vi "spike_data_packete.vi"(8 "Log File in":refnum<k34>, 11 "data out":string) -> (3 "output cluster":T1)   [LabVIEW 2017]
uses:
  Control 2.ctl
panel:
  out "data":string
  in  "?":T1
  out "DIN":string
  out "DEV":string
  out "RES":string
  out "LEN":string
  out "SYNC":string
  out "CMD":string
  out "A(I16) 11":i16
  out "Received Data 4":dbl[](graph)
  out "Received Data 3":T2(graph)
  out "BR4_5 (bending Y) 5":string
  out "BR3_5 (bending X) 5":string
  out "BR4_7 (bending Y) 7":string
  out "BR3_7 (bending X) 7":string
  out "BR2_7 (torsion)6 2":string
  out "BR1_7 (axial_force_ 7":string
  out "BR4_6 (bending Y) 6":string
  out "BR3_6 (bending X) 6":string
  out "BR2_6 (torsion)6":string
  out "BR1_6 (axial_force_ 6":string
  out "BR2_5 (torsion) 5":string
  out "BR1_5 (axial_force_ 5":string
  out "BR4_4 (bending Y) 4":string
  out "BR3_4 (bending X) 4":string
  out "BR2_4 (torsion) 4":string
  out "BR1_4 (axial_force_ 4":string
  out "BR4_3 (bending Y) 3":string
  out "BR3_3 (bending X) 3":string
  out "BR2_3 (torsion) 3":string
  out "BR1_3 (axial_force_ 3":string
  out "BR4_2 (bending Y) 2":string
  out "BR3_2 (bending X) 2":string
  out "RSSI":string
  out "PKT":string
  out "SPEF":string
  out "SPER":string
  out "BR2_2 (torsion) 2":string
  out "BR1_2 (axial_force_ 2":string
  out "BR4_1 (bending Y)":string
  out "BR3_1 (bending X)":string
  out "BR2_1 (torsion)":string
  out "BR1_1 (axial_force_":string
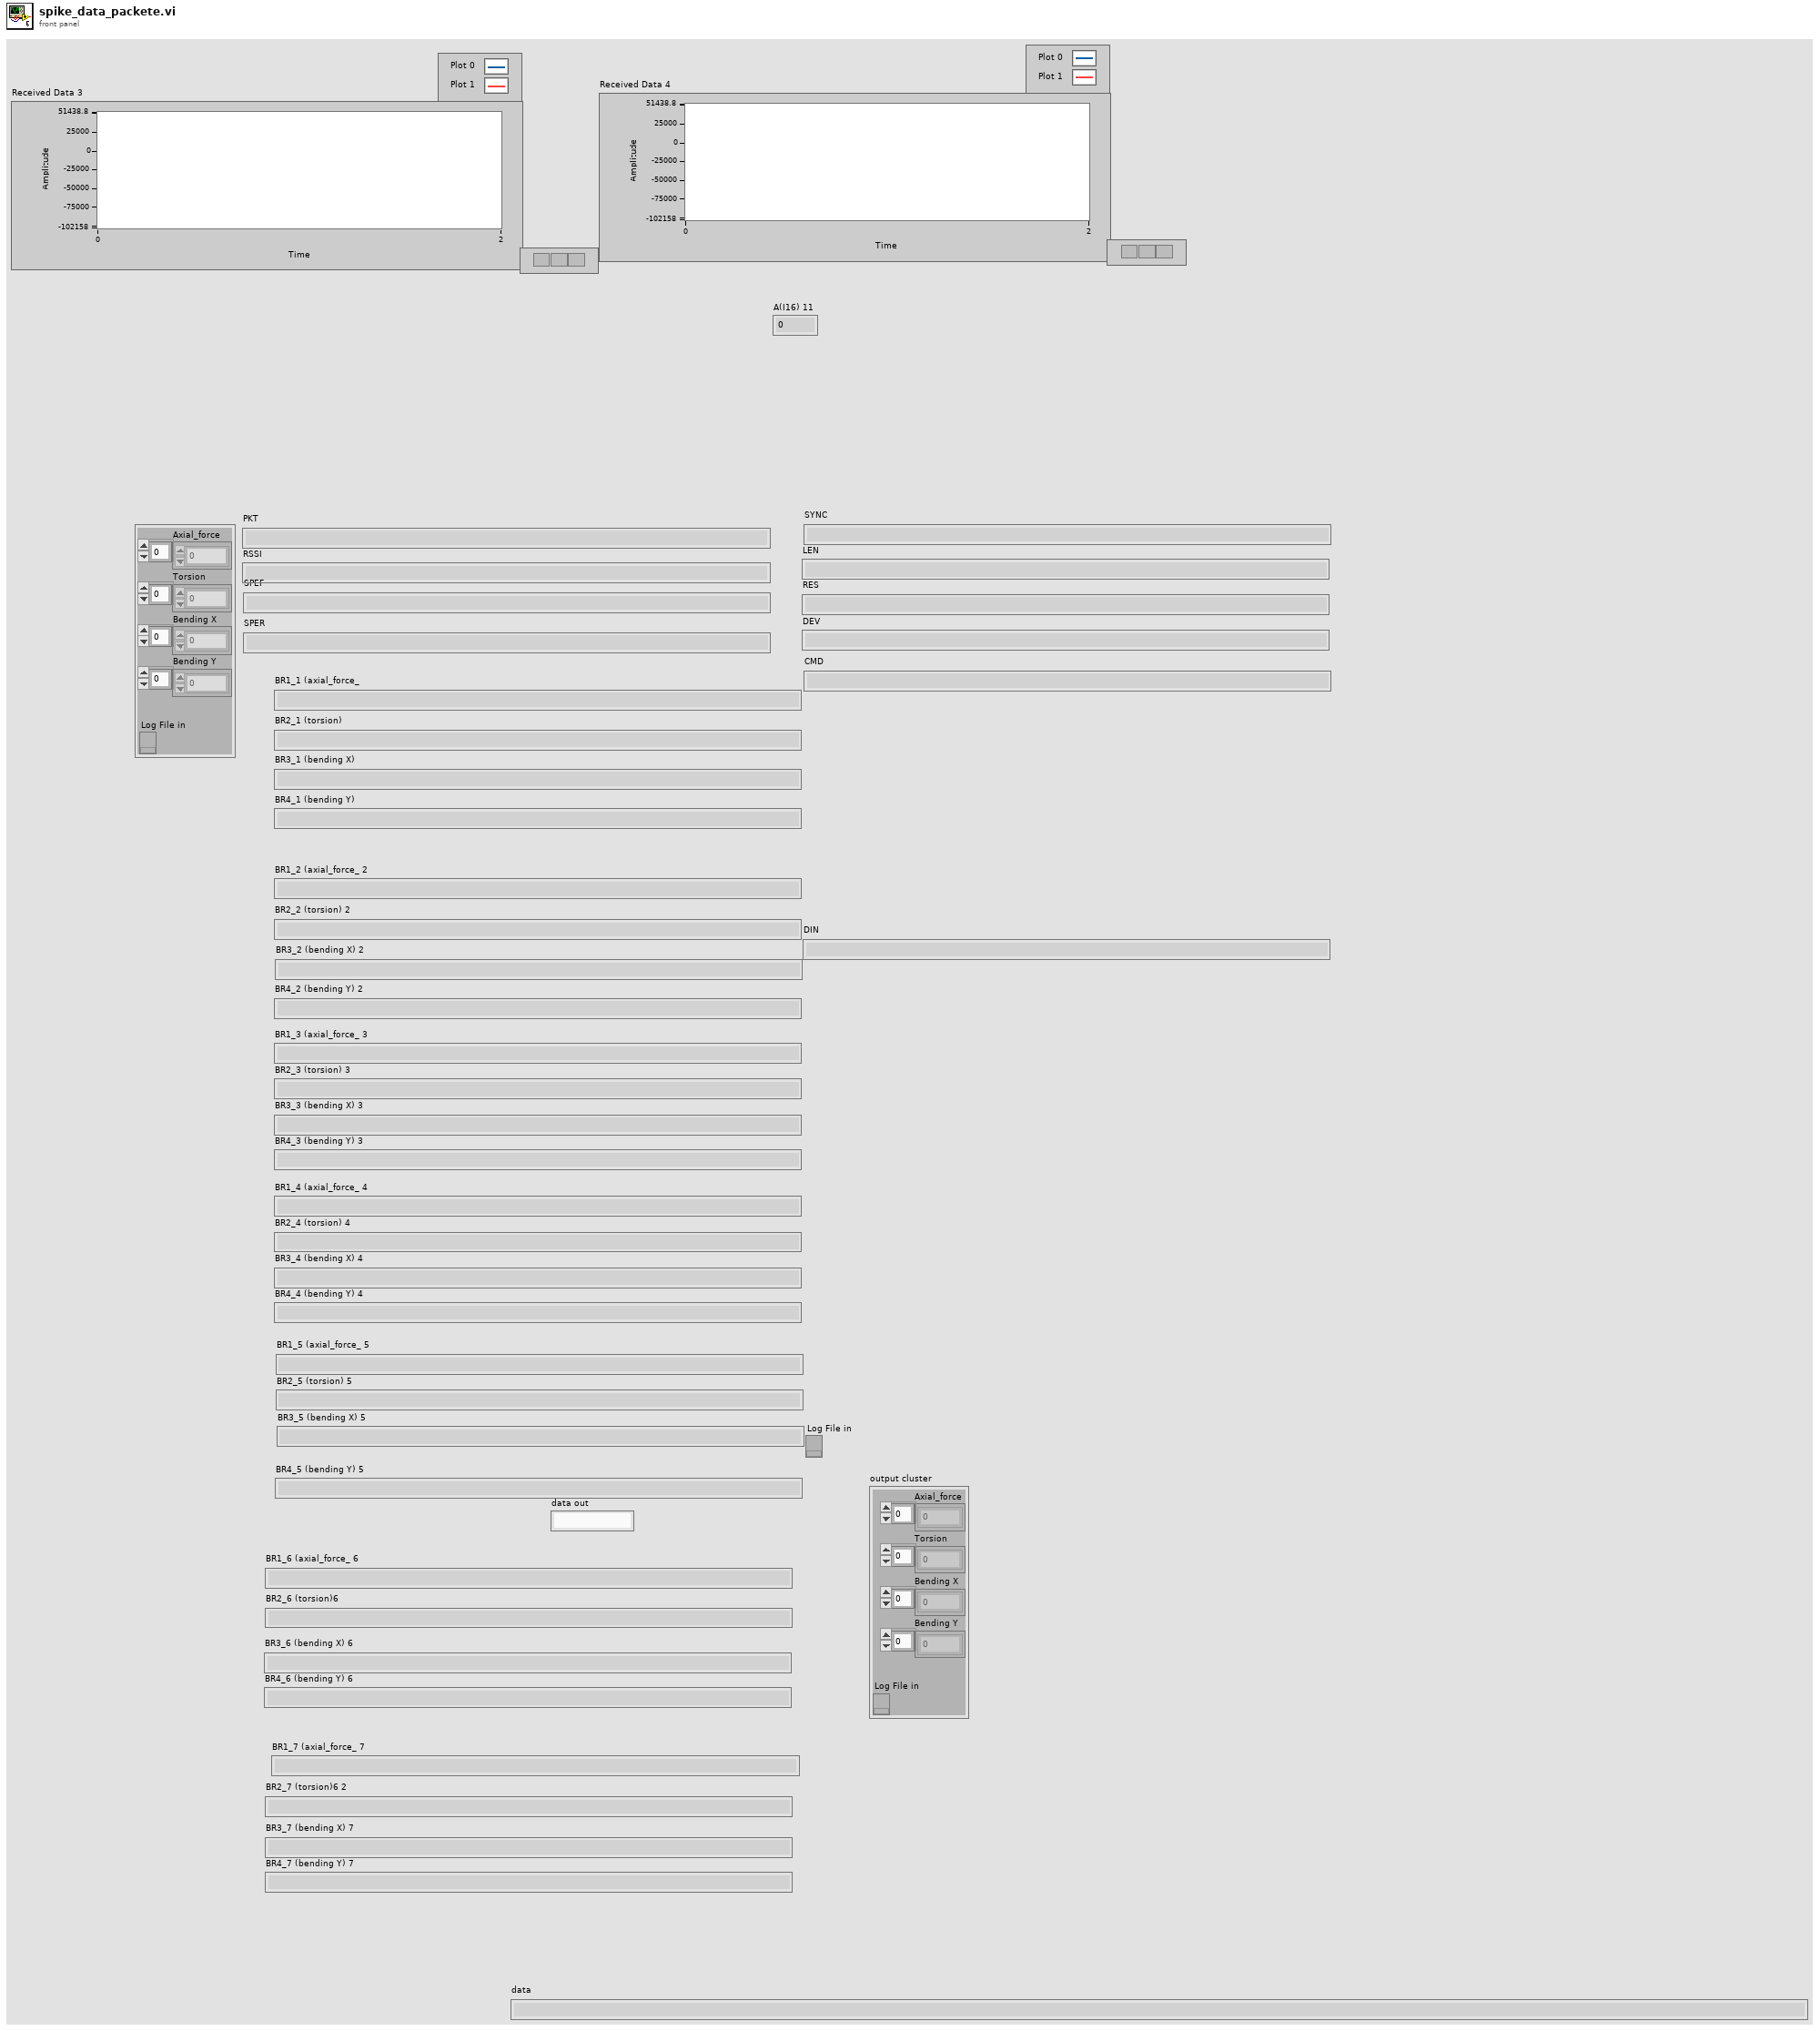
[diagram p1: front panel]
types:
  T1 = typedef "Control 2.ctl" = cluster{"Axial_force":i16[], "Torsion":i16[], "Bending X":i16[], "Bending Y":i16[], "Log File in":refnum<k34>}
  T2 = cluster{"[0]":i16, "[1]":i16, "[2]":i16, "[3]":i16, "[4]":i16, "[5]":i16, "[6]":i16, "[7]":i16, "[8]":i16}
  T3 = enum16{"big-endian, network order", "native, host order", "little-endian"}
  T4 = cluster{"A(I16)":i16, "A(I8) 2":i8, "A(I8) 3":i8, "A(I18) 4":i8, "A(I8) 5":i8, "A(I8) 6":i8, "A(I16) 7":i16, "A(I8) 8":i8, "A(I8) 9":i8, "A(I16) 10":i16, "A(I16) 11":i16, "A(I16) 12":i16, "A(I16) 13":i16, "A(I16) 14":i16, "A(I16) 15":i16, "A(I16) 16":i16, "A(I16) 17":i16, "A(I16) 18":i16, "A(I16) 19":i16, "A(I16) 20":i16, "A(I16) 21":i16, "A(I16) 22":i16, "A(I16) 23":i16, "A(I16) 24":i16, "A(I16) 25":i16, "A(I16) 26":i16, "A(I16) 27":i16, "A(I16) 28":i16, "A(I16) 29":i16, "A(I16) 30":i16, "A(I16) 31":i16, "A(I16) 32":i16, "A(I16) 33":i16, "A(I16) 34":i16, "A(I16) 35":i16, "A(I16) 36":i16, "A(I16) 37":i16, "A(I16) 38":i16, "A(I16) 39":i16, "A(I16) 40":i16, "A(I16) 41":i16, "A(I16) 42":i16, "A(I16) 43":i16, "A(I16) 44":i16, "A(I16) 45":i16, "A(I16) 46":i16, "A(I16) 47":i16, "A(I16) 48":i16, "A(I16) 49":i16, "A(I16) 50":i16, "A(I16) 51":i16, "A(I16) 52":i16, "A(I16) 53":i16, "A(I16) 54":i16, "A(I16) 55":i16, "A(I16) 56":i16, "A(I16) 57":i16, "A(I16) 58":i16, "A(I16) 59":i16, "A(I16) 60":i16, "A(I16) 61":i16, "A(I16) 62":i16, "A(I16) 63":i16, "A(I16) 64":i16, "A(I16) 65":i16, "A(I16) 66":i16, "A(I16) 67":i16, "A(I16) 68":i16, "A(I16) 69":i16, "A(I16) 70":i16}
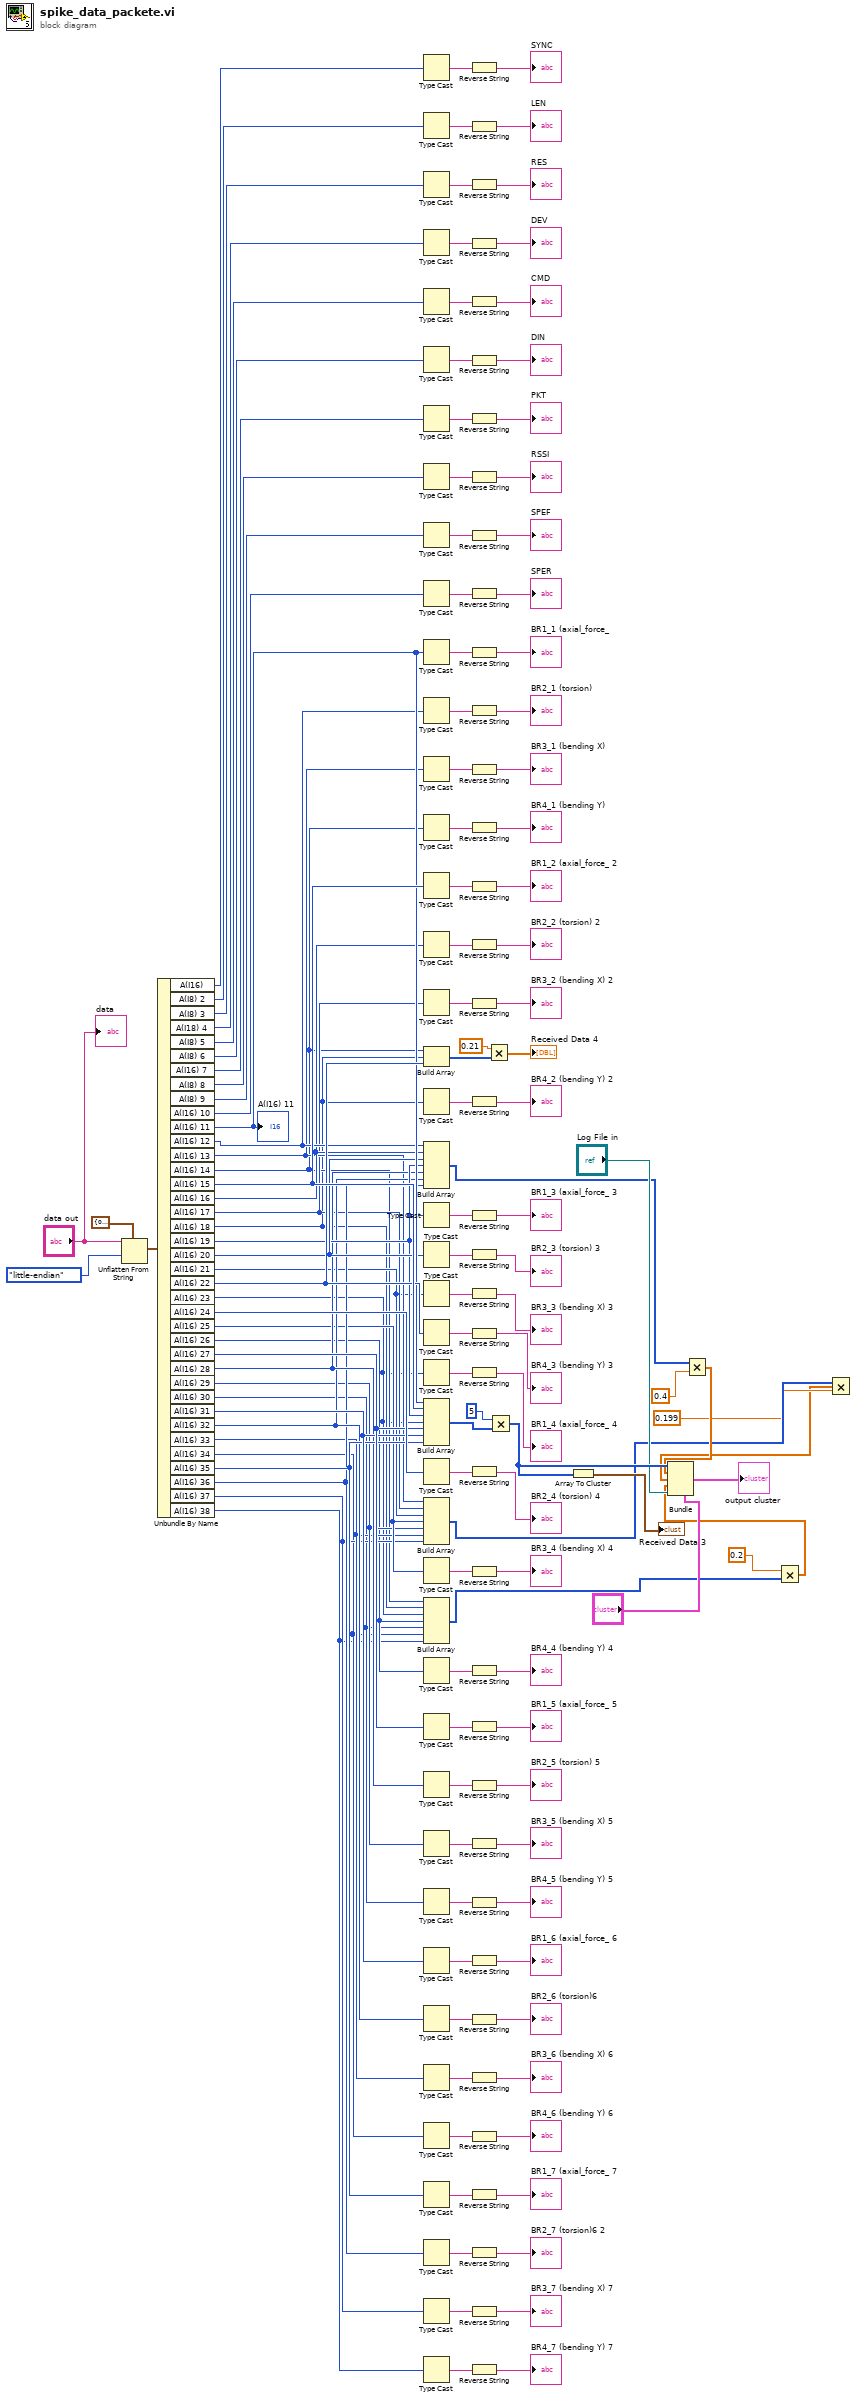
[diagram p0: block diagram]
diagram:
  n1 = Unflatten From String(type=T4 {"A(I16)"=0, "A(I8) 2"=0, "A(I8) 3"=0, "A(I18) 4"=0, "A(I8) 5"=0, "A(I8) 6"=0, "A(I16) 7"=0, "A(I8) 8"=0, "A(I8) 9"=0, "A(I16) 10"=0, "A(I16) 11"=0, "A(I16) 12"=0, "A(I16) 13"=0, "A(I16) 14"=0, "A(I16) 15"=0, "A(I16) 16"=0, "A(I16) 17"=0, "A(I16) 18"=0, "A(I16) 19"=0, "A(I16) 20"=0, "A(I16) 21"=0, "A(I16) 22"=0, "A(I16) 23"=0, "A(I16) 24"=0, "A(I16) 25"=0, "A(I16) 26"=0, "A(I16) 27"=0, "A(I16) 28"=0, "A(I16) 29"=0, "A(I16) 30"=0, "A(I16) 31"=0, "A(I16) 32"=0, "A(I16) 33"=0, "A(I16) 34"=0, "A(I16) 35"=0, "A(I16) 36"=0, "A(I16) 37"=0, "A(I16) 38"=0, "A(I16) 39"=0, "A(I16) 40"=0, "A(I16) 41"=0, "A(I16) 42"=0, "A(I16) 43"=0, "A(I16) 44"=0, "A(I16) 45"=0, "A(I16) 46"=0, "A(I16) 47"=0, "A(I16) 48"=0, "A(I16) 49"=0, "A(I16) 50"=0, "A(I16) 51"=0, "A(I16) 52"=0, "A(I16) 53"=0, "A(I16) 54"=0, "A(I16) 55"=0, "A(I16) 56"=0, "A(I16) 57"=0, "A(I16) 58"=0, "A(I16) 59"=0, "A(I16) 60"=0, "A(I16) 61"=0, "A(I16) 62"=0, "A(I16) 63"=0, "A(I16) 64"=0, "A(I16) 65"=0, "A(I16) 66"=0, "A(I16) 67"=0, "A(I16) 68"=0, "A(I16) 69"=0, "A(I16) 70"=0}, binary string="data out", byte order (0:big-endian, network order)=T3."little-endian") -> (value=w54:T4)  [unwired: 2 in, 2 out]
  n2 = Unbundle By Name(w54) -> ("A(I16)"=w43:i16, "A(I8) 2"=w42:i8, "A(I8) 3"=w41:i8, "A(I18) 4"=w40:i8, "A(I8) 5"=w39:i8, "A(I8) 6"=w38:i8, "A(I16) 7"=w132:i16, "A(I8) 8"=w135:i8, "A(I8) 9"=w134:i8, "A(I16) 10"=w133:i16, "A(I16) 11"=w55:i16, "A(I16) 12"=w31:i16, "A(I16) 13"=w24:i16, "A(I16) 14"=w17:i16, "A(I16) 15"=w67:i16, "A(I16) 16"=w30:i16, "A(I16) 17"=w23:i16, "A(I16) 18"=w16:i16, "A(I16) 19"=w28:i16, "A(I16) 20"=w29:i16, "A(I16) 21"=w22:i16, "A(I16) 22"=w60:i16, "A(I16) 23"=w15:i16, "A(I16) 24"=w87:i16, "A(I16) 25"=w21:i16, "A(I16) 26"=w14:i16, "A(I16) 27"=w63:i16, "A(I16) 28"=w27:i16, "A(I16) 29"=w20:i16, "A(I16) 30"=w13:i16, "A(I16) 31"=w62:i16, "A(I16) 32"=w26:i16, "A(I16) 33"=w19:i16, "A(I16) 34"=w12:i16, "A(I16) 35"=w61:i16, "A(I16) 36"=w25:i16, "A(I16) 37"=w18:i16, "A(I16) 38"=w11:i16)
  "A(I16) 11" <- w55
  n3 = Type Cast(x=w43) -> (*(type *) &x=w49:string)  [unwired: 1 in]
  n4 = Type Cast(x=w42) -> (*(type *) &x=w53:string)  [unwired: 1 in]
  n5 = Type Cast(x=w41) -> (*(type *) &x=w52:string)  [unwired: 1 in]
  n6 = Type Cast(x=w40) -> (*(type *) &x=w51:string)  [unwired: 1 in]
  n7 = Type Cast(x=w39) -> (*(type *) &x=w50:string)  [unwired: 1 in]
  n8 = Type Cast(x=w38) -> (*(type *) &x=w37:string)  [unwired: 1 in]
  n9 = Type Cast(x=w132) -> (*(type *) &x=w131:string)  [unwired: 1 in]
  n10 = Type Cast(x=w135) -> (*(type *) &x=w130:string)  [unwired: 1 in]
  n11 = Type Cast(x=w134) -> (*(type *) &x=w127:string)  [unwired: 1 in]
  n12 = Type Cast(x=w133) -> (*(type *) &x=w128:string)  [unwired: 1 in]
  n13 = Type Cast(x=w55) -> (*(type *) &x=w129:string)  [unwired: 1 in]
  n14 = Type Cast(x=w31) -> (*(type *) &x=w126:string)  [unwired: 1 in]
  n15 = Type Cast(x=w24) -> (*(type *) &x=w124:string)  [unwired: 1 in]
  n16 = Type Cast(x=w17) -> (*(type *) &x=w122:string)  [unwired: 1 in]
  n17 = Type Cast(x=w67) -> (*(type *) &x=w120:string)  [unwired: 1 in]
  n18 = Type Cast(x=w30) -> (*(type *) &x=w118:string)  [unwired: 1 in]
  n19 = Type Cast(x=w23) -> (*(type *) &x=w111:string)  [unwired: 1 in]
  n20 = Build Array(w17, w16, w60) -> (w58:i16[])
  n21 = Type Cast(x=w16) -> (*(type *) &x=w112:string)  [unwired: 1 in]
  n22 = Build Array(w31, w30, w29, w28, w27, w26, w25) -> (w9:i16[])
  n23 = Type Cast(x=w28) -> (*(type *) &x=w108:string)  [unwired: 1 in]
  n24 = Type Cast(x=w29) -> (*(type *) &x=w106:string)  [unwired: 1 in]
  n25 = Type Cast(x=w22) -> (*(type *) &x=w104:string)  [unwired: 1 in]
  n26 = Type Cast(x=w60) -> (*(type *) &x=w102:string)  [unwired: 1 in]
  n27 = Type Cast(x=w15) -> (*(type *) &x=w93:string)  [unwired: 1 in]
  n28 = Build Array(w55, w67, w28, w15, w63, w62, w61) -> (w65:i16[])
  n29 = Type Cast(x=w87) -> (*(type *) &x=w95:string)  [unwired: 1 in]
  n30 = Build Array(w24, w23, w22, w21, w20, w19, w18) -> (w6:i16[])
  n31 = Type Cast(x=w21) -> (*(type *) &x=w97:string)  [unwired: 1 in]
  n32 = Build Array(w17, w16, w15, w14, w13, w12, w11) -> (w3:i16[])
  n33 = Type Cast(x=w14) -> (*(type *) &x=w99:string)  [unwired: 1 in]
  n34 = Type Cast(x=w63) -> (*(type *) &x=w92:string)  [unwired: 1 in]
  n35 = Type Cast(x=w27) -> (*(type *) &x=w90:string)  [unwired: 1 in]
  n36 = Type Cast(x=w20) -> (*(type *) &x=w71:string)  [unwired: 1 in]
  n37 = Type Cast(x=w13) -> (*(type *) &x=w69:string)  [unwired: 1 in]
  n38 = Type Cast(x=w62) -> (*(type *) &x=w88:string)  [unwired: 1 in]
  n39 = Type Cast(x=w26) -> (*(type *) &x=w80:string)  [unwired: 1 in]
  n40 = Type Cast(x=w19) -> (*(type *) &x=w84:string)  [unwired: 1 in]
  n41 = Type Cast(x=w12) -> (*(type *) &x=w83:string)  [unwired: 1 in]
  n42 = Type Cast(x=w61) -> (*(type *) &x=w72:string)  [unwired: 1 in]
  n43 = Type Cast(x=w25) -> (*(type *) &x=w79:string)  [unwired: 1 in]
  n44 = Type Cast(x=w18) -> (*(type *) &x=w75:string)  [unwired: 1 in]
  n45 = Type Cast(x=w11) -> (*(type *) &x=w76:string)  [unwired: 1 in]
  n46 = Reverse String(1:w49) -> (0:→"SYNC":string)
  n47 = Reverse String(1:w53) -> (0:→"LEN":string)
  n48 = Reverse String(1:w52) -> (0:→"RES":string)
  n49 = Reverse String(1:w51) -> (0:→"DEV":string)
  n50 = Reverse String(1:w50) -> (0:→"CMD":string)
  n51 = Reverse String(1:w37) -> (0:→"DIN":string)
  n52 = Reverse String(1:w131) -> (0:→"PKT":string)
  n53 = Reverse String(1:w130) -> (0:→"RSSI":string)
  n54 = Reverse String(1:w127) -> (0:→"SPEF":string)
  n55 = Reverse String(1:w128) -> (0:→"SPER":string)
  n56 = Reverse String(1:w129) -> (0:→"BR1_1 (axial_force_":string)
  n57 = Reverse String(1:w126) -> (0:→"BR2_1 (torsion)":string)
  n58 = Reverse String(1:w124) -> (0:→"BR3_1 (bending X)":string)
  n59 = Reverse String(1:w122) -> (0:→"BR4_1 (bending Y)":string)
  n60 = Reverse String(1:w120) -> (0:→"BR1_2 (axial_force_ 2":string)
  n61 = Reverse String(1:w118) -> (0:→"BR2_2 (torsion) 2":string)
  n62 = Reverse String(1:w111) -> (0:→"BR3_2 (bending X) 2":string)
  n63 = Reverse String(1:w112) -> (0:→"BR4_2 (bending Y) 2":string)
  n64 = Reverse String(1:w108) -> (0:→"BR1_3 (axial_force_ 3":string)
  n65 = Reverse String(1:w106) -> (0:→"BR2_3 (torsion) 3":string)
  n66 = Reverse String(1:w104) -> (0:→"BR3_3 (bending X) 3":string)
  n67 = Reverse String(1:w102) -> (0:→"BR4_3 (bending Y) 3":string)
  n68 = Reverse String(1:w93) -> (0:→"BR1_4 (axial_force_ 4":string)
  n69 = Reverse String(1:w95) -> (0:→"BR2_4 (torsion) 4":string)
  n70 = Reverse String(1:w97) -> (0:→"BR3_4 (bending X) 4":string)
  n71 = Reverse String(1:w99) -> (0:→"BR4_4 (bending Y) 4":string)
  n72 = Reverse String(1:w92) -> (0:→"BR1_5 (axial_force_ 5":string)
  n73 = Reverse String(1:w90) -> (0:→"BR2_5 (torsion) 5":string)
  n74 = Reverse String(1:w71) -> (0:→"BR3_5 (bending X) 5":string)
  n75 = Reverse String(1:w69) -> (0:→"BR4_5 (bending Y) 5":string)
  n76 = Reverse String(1:w88) -> (0:→"BR1_6 (axial_force_ 6":string)
  n77 = Reverse String(1:w80) -> (0:→"BR2_6 (torsion)6":string)
  n78 = Reverse String(1:w84) -> (0:→"BR3_6 (bending X) 6":string)
  n79 = Reverse String(1:w83) -> (0:→"BR4_6 (bending Y) 6":string)
  n80 = Reverse String(1:w72) -> (0:→"BR1_7 (axial_force_ 7":string)
  n81 = Reverse String(1:w79) -> (0:→"BR2_7 (torsion)6 2":string)
  n82 = Reverse String(1:w75) -> (0:→"BR3_7 (bending X) 7":string)
  n83 = Reverse String(1:w76) -> (0:→"BR4_7 (bending Y) 7":string)
  n84 = Multiply(x=0.21, y=w58) -> (x*y=→"Received Data 4":dbl[])
  n85 = Multiply(x=i16 5, y=w65) -> (x*y=w35:i16[])
  n86 = Array To Cluster(array=w35) -> (cluster=→"Received Data 3":T2)
  n87 = Multiply(x=w9, y=0.4) -> (x*y=w8:dbl[])
  n88 = Multiply(x=0.2, y=w3) -> (x*y=w1:dbl[])
  n89 = Multiply(x=w6, y=0.199) -> (x*y=w4:dbl[])
  n90 = Bundle(cluster="?", "Axial_force"=w35, "Torsion"=w8, "Bending X"=w4, "Bending Y"=w1, "Log File in"="Log File in") -> (→"output cluster":T1)
  "data" <- "data out"
